vi "S2C_VLFT10_Proc_Read-WriteScales.vi"(8 "Error In":errorcluster, 10 "ScaleAction":u16(ring) items=["Read", "Write"], 11 "ScaleType":u16(ring) items=["Voltage", "Current"]) -> (0 "Error Out":errorcluster, 3 "Pass?":bool)   [LabVIEW 2015]
uses:
  Fornax/VIs/PolyDriver/S2C_FORNAX_Poly_ViperCmd.vi
panel:
  out "CurrSensScales":T1
  out "VoltSensScales":T2
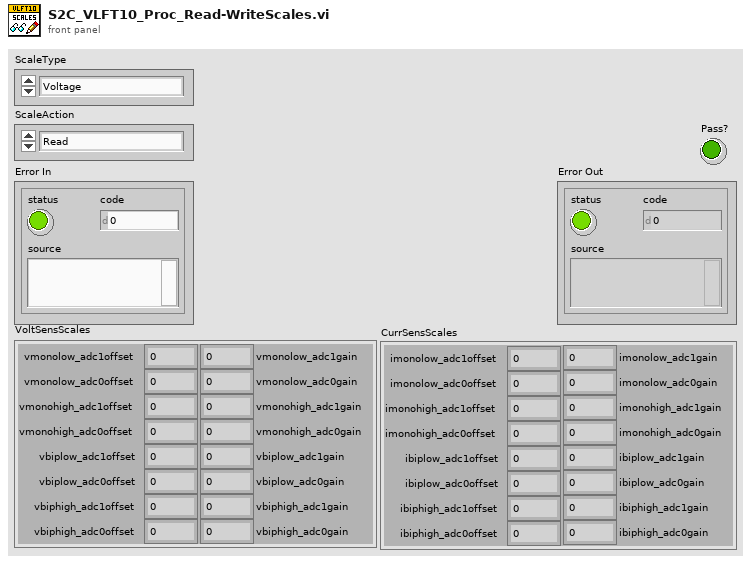
[diagram p1: front panel]
types:
  T1 = cluster{"imonolow_adc1offset":dbl, "imonolow_adc1gain":dbl, "imonolow_adc0offset":dbl, "imonolow_adc0gain":dbl, "imonohigh_adc1offset":dbl, "imonohigh_adc1gain":dbl, "imonohigh_adc0offset":dbl, "imonohigh_adc0gain":dbl, "ibiplow_adc1offset":dbl, "ibiplow_adc1gain":dbl, "ibiplow_adc0offset":dbl, "ibiplow_adc0gain":dbl, "ibiphigh_adc1offset":dbl, "ibiphigh_adc1gain":dbl, "ibiphigh_adc0offset":dbl, "ibiphigh_adc0gain":dbl}
  T2 = cluster{"vmonolow_adc1offset":dbl, "vmonolow_adc1gain":dbl, "vmonolow_adc0offset":dbl, "vmonolow_adc0gain":dbl, "vmonohigh_adc1offset":dbl, "vmonohigh_adc1gain":dbl, "vmonohigh_adc0offset":dbl, "vmonohigh_adc0gain":dbl, "vbiplow_adc1offset":dbl, "vbiplow_adc1gain":dbl, "vbiplow_adc0offset":dbl, "vbiplow_adc0gain":dbl, "vbiphigh_adc1offset":dbl, "vbiphigh_adc1gain":dbl, "vbiphigh_adc0offset":dbl, "vbiphigh_adc0gain":dbl}
  T3 = cluster{"Partition":string, "Message":string, "M_ViperMessage":string, "M_SrcId":i32}
  T4 = cluster{"vmonolow_adc0gain":dbl, "vmonolow_adc0offset":dbl, "vmonolow_adc1gain":dbl, "vmonolow_adc1offset":dbl, "vmonohigh_adc0gain":dbl, "vmonohigh_adc0offset":dbl, "vmonohigh_adc1gain":dbl, "vmonohigh_adc1offset":dbl, "vbiplow_adc0gain":dbl, "vbiplow_adc0offset":dbl, "vbiplow_adc1gain":dbl, "vbiplow_adc1offset":dbl, "vbiphigh_adc0gain":dbl, "vbiphigh_adc0offset":dbl, "vbiphigh_adc1gain":dbl, "vbiphigh_adc1offset":dbl}
  T5 = cluster{"Partition":string, "Message":string, "M_destId":i32, "M_message":string, "M_Crc32":i32}
  T6 = cluster{"imonolow_adc0gain":dbl, "imonolow_adc0offset":dbl, "imonolow_adc1gain":dbl, "imonolow_adc1offset":dbl, "imonohigh_adc0gain":dbl, "imonohigh_adc0offset":dbl, "imonohigh_adc1gain":dbl, "imonohigh_adc1offset":dbl, "ibiplow_adc0gain":dbl, "ibiplow_adc0offset":dbl, "ibiplow_adc1gain":dbl, "ibiplow_adc1offset":dbl, "ibiphigh_adc0gain":dbl, "ibiphigh_adc0offset":dbl, "ibiphigh_adc1gain":dbl, "ibiphigh_adc1offset":dbl}
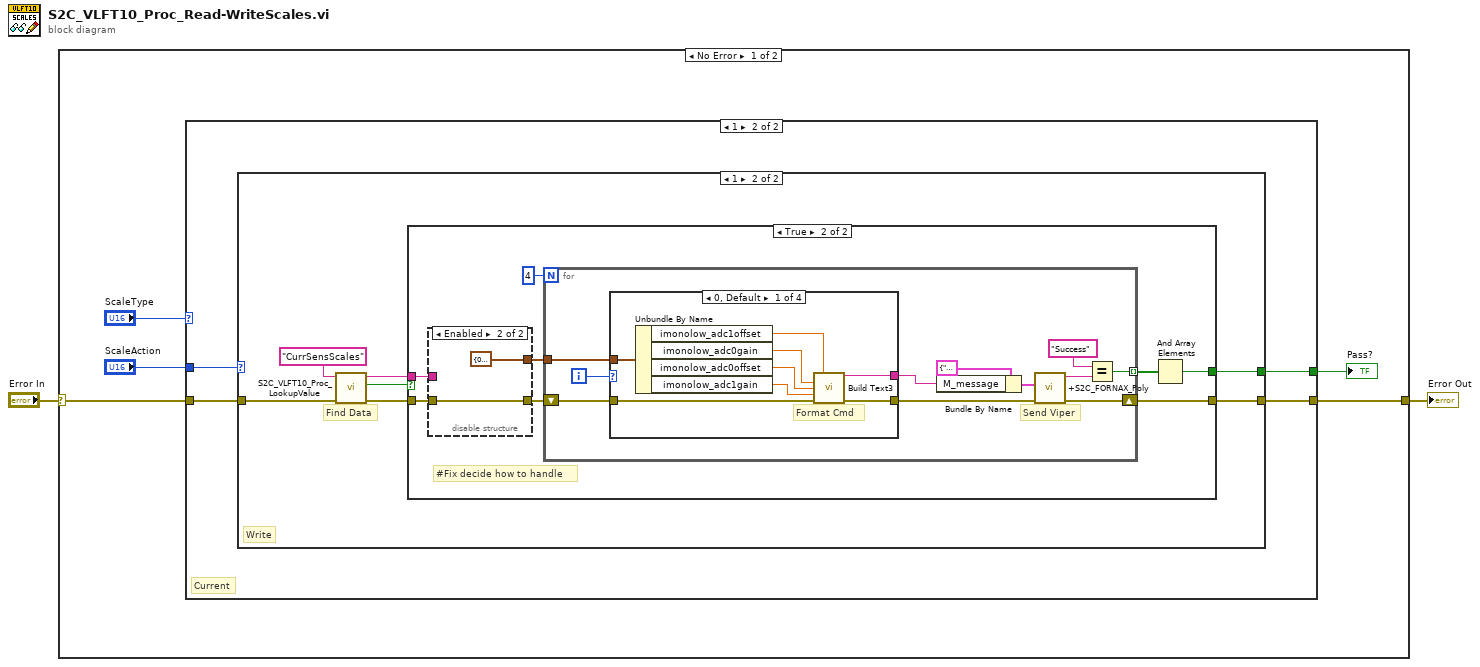
[diagram p0: block diagram]
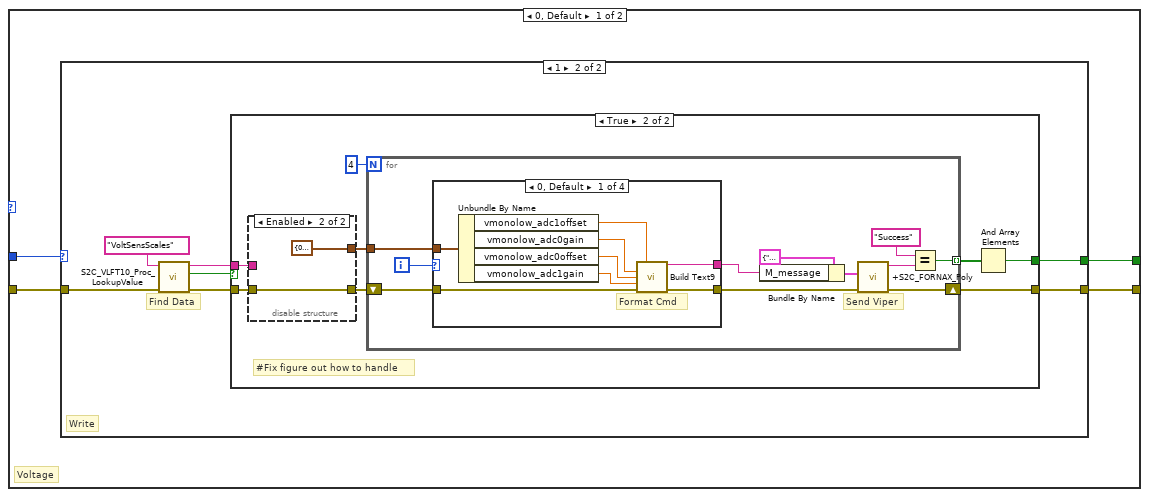
[diagram p2: hidden frame]
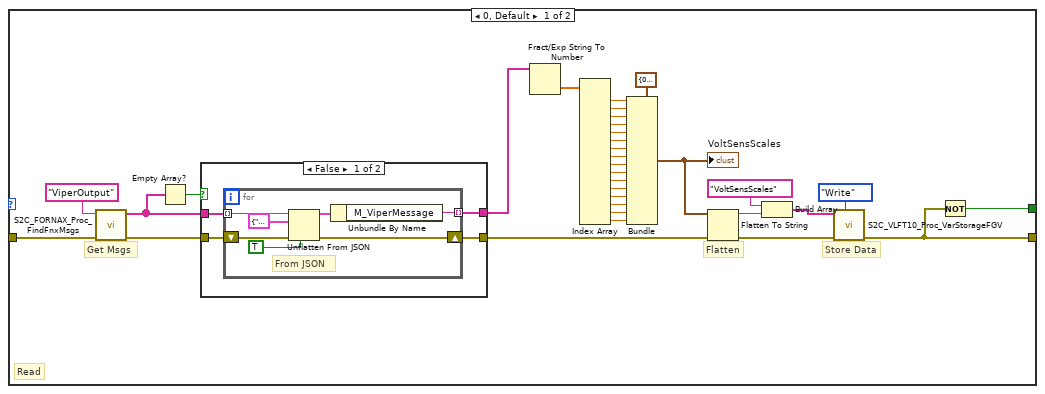
[diagram p3: hidden frame]
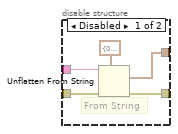
[diagram p6: hidden frame]
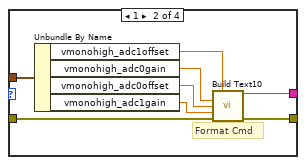
[diagram p7: hidden frame]
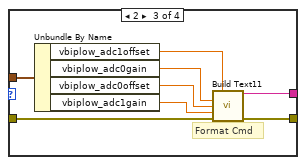
[diagram p8: hidden frame]
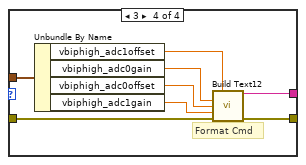
[diagram p9: hidden frame]
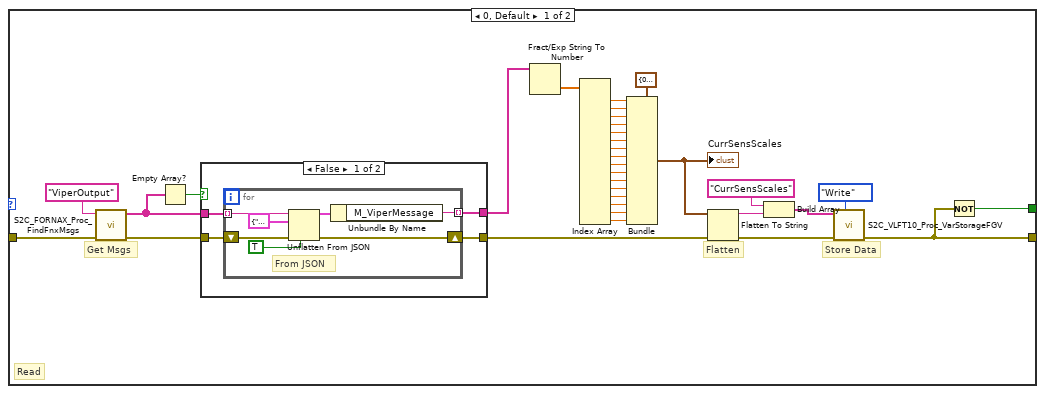
[diagram p10: hidden frame]
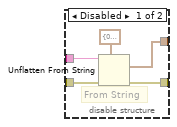
[diagram p13: hidden frame]
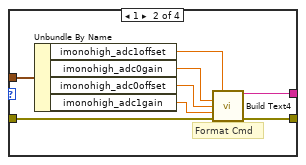
[diagram p14: hidden frame]
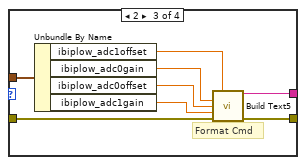
[diagram p15: hidden frame]
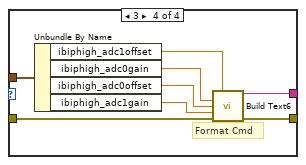
[diagram p16: hidden frame]
diagram:
  n1 = case shown="No Error" "Error In" {
    selector: "Error In" -> [w4 w238]
    tunnel: [w7 w238] -> w1
    frame No Error {
      n2 = case shown="1" "ScaleType" {
        tunnel: w4 -> [w11 w126]
        tunnel: [w10 w125] -> w7
        tunnel: "ScaleAction" -> [w9 w124]
        tunnel: [w8 w123] -> w3
        frame 0, Default {
          # "Voltage"
          n3 = case shown="1" w9 {
            tunnel: w11 -> [w14 w60]
            tunnel: [w13 w63] -> w10
            tunnel: [w12 w62] -> w8
            frame 0, Default {
              # "Flatten"
              # "Store Data"
              # "Read"
              # "Get Msgs"
              n4 = call "S2C_FORNAX_Proc_FindFnxMsgs.vi"("Error In"=w14, "MsgName"="ViperOutput") -> ("Error Out"=w43:errorcluster, "Messages"=w42:string[])  [unwired: 8 in]
              n5 = Empty Array?(array=w42) -> (empty?=w41:bool)
              n6 = case shown="False" w41 {
                tunnel: w43 -> [w48 w56]
                tunnel: w42 -> [w47 _]
                tunnel: [w45 w56] -> w15
                tunnel: [w46 _] -> w31
                frame False {
                  n7 = for {
                    tunnel: w47 -> [w52] mode=indexing
                    tunnel: [w50] -> w46 mode=indexing
                    shift-right: [w49] -> w45
                    shift-left: w48 -> [w54]
                    # "From JSON"
                    n8 = Unflatten From JSON(JSON string=w52, type and defaults=T3 {"Partition"="", "Message"="", "M_ViperMessage"="", "M_SrcId"=0}, default null elements? (F)=TRUE, error in (no error)=w54) -> (value=w51:T3, error out=w49:errorcluster)  [unwired: 3 in]
                    n9 = Unbundle By Name(w51) -> ("M_ViperMessage"=w50:string)
                  }
                }
                frame True {
                }
              }
              n10 = Fract/Exp String To Number(string=w31) -> (number=w40:dbl[])  [unwired: 3 in, 1 out]
              n11 = Index Array(array=w40) -> (element #1=w39:dbl, element #2=w38:dbl, element #3=w37:dbl, element #4=w36:dbl, element #5=w35:dbl, element #6=w34:dbl, element #7=w33:dbl, element #8=w32:dbl, element #9=w29:dbl, element #10=w28:dbl, element #11=w27:dbl, element #12=w26:dbl, element #13=w25:dbl, element #14=w24:dbl, element #15=w23:dbl, element #16=w22:dbl)  [unwired: 16 in]
              n12 = Bundle(cluster=T2 {"vmonolow_adc1offset"=0.0, "vmonolow_adc1gain"=0.0, "vmonolow_adc0offset"=0.0, "vmonolow_adc0gain"=0.0, "vmonohigh_adc1offset"=0.0, "vmonohigh_adc1gain"=0.0, "vmonohigh_adc0offset"=0.0, "vmonohigh_adc0gain"=0.0, "vbiplow_adc1offset"=0.0, "vbiplow_adc1gain"=0.0, "vbiplow_adc0offset"=0.0, "vbiplow_adc0gain"=0.0, "vbiphigh_adc1offset"=0.0, "vbiphigh_adc1gain"=0.0, "vbiphigh_adc0offset"=0.0, "vbiphigh_adc0gain"=0.0} ("VoltSensScales"), "vmonolow_adc1offset"=w39, "vmonolow_adc1gain"=w38, "vmonolow_adc0offset"=w37, "vmonolow_adc0gain"=w36, "vmonohigh_adc1offset"=w35, "vmonohigh_adc1gain"=w34, "vmonohigh_adc0offset"=w33, "vmonohigh_adc0gain"=w32, "vbiplow_adc1offset"=w29, "vbiplow_adc1gain"=w28, "vbiplow_adc0offset"=w27, "vbiplow_adc0gain"=w26, "vbiphigh_adc1offset"=w25, "vbiphigh_adc1gain"=w24, "vbiphigh_adc0offset"=w23, "vbiphigh_adc0gain"=w22) -> (w20:T2)
              "VoltSensScales" <- w20
              n13 = Flatten To String(anything=w20, error in (no error)=w15) -> (data string=w19:string, error out=w16:errorcluster)  [unwired: 2 in, 1 out]
              n14 = Build Array("VoltSensScales", w19) -> (w17:string[])
              n15 = call "S2C_VLFT10_Proc_VarStorageFGV.vi"("Action"=enum16{"Read", "Write", "Clear"}."Write", "Error In"=w16, "Data In"=w17) -> ("Error Out"=w13:errorcluster)  [unwired: 7 in, 1 out]
              n16 = Not(x=w13) -> (.not. x?=w12:bool)
            }
            frame 1 {
              # "Write"
              # "Find Data"
              n17 = call "S2C_VLFT10_Proc_LookupValue.vi"("Error In"=w60, "VarName"="VoltSensScales") -> ("Error Out"=w59:errorcluster, "Found?"=w57:bool, "VarValue"=w58:string)  [unwired: 7 in]
              n18 = case shown="True" w57 {
                tunnel: w58 -> [_ w67]
                tunnel: w59 -> [w64 w68]
                tunnel: [w64 w65] -> w63
                tunnel: [_ w72] -> w62
                frame False {
                }
                frame True {
                  # "#Fix figure out how to handle"
                  n19 = disable-structure shown="Enabled" {
                    disable-tunnel: [w77 w79] -> w70
                    disable-tunnel: [w76 T2 {"vmonolow_adc1offset"=0.0, "vmonolow_adc1gain"=1.0, "vmonolow_adc0offset"=0.0, "vmonolow_adc0gain"=1.0, "vmonohigh_adc1offset"=0.0, "vmonohigh_adc1gain"=1.0, "vmonohigh_adc0offset"=0.0, "vmonohigh_adc0gain"=1.0, "vbiplow_adc1offset"=0.0, "vbiplow_adc1gain"=1.0, "vbiplow_adc0offset"=0.0, "vbiplow_adc0gain"=1.0, "vbiphigh_adc1offset"=0.0, "vbiphigh_adc1gain"=1.0, "vbiphigh_adc0offset"=0.0, "vbiphigh_adc0gain"=1.0} ("VoltSensScales 2")] -> w69
                    disable-tunnel: w68 -> [w75 w79]
                    disable-tunnel: w67 -> [w74 _]
                    frame Disabled {
                      # "From String"
                      n20 = Unflatten From String(type=T4 {"vmonolow_adc0gain"=0.0, "vmonolow_adc0offset"=0.0, "vmonolow_adc1gain"=0.0, "vmonolow_adc1offset"=0.0, "vmonohigh_adc0gain"=0.0, "vmonohigh_adc0offset"=0.0, "vmonohigh_adc1gain"=0.0, "vmonohigh_adc1offset"=0.0, "vbiplow_adc0gain"=0.0, "vbiplow_adc0offset"=0.0, "vbiplow_adc1gain"=0.0, "vbiplow_adc1offset"=0.0, "vbiphigh_adc0gain"=0.0, "vbiphigh_adc0offset"=0.0, "vbiphigh_adc1gain"=0.0, "vbiphigh_adc1offset"=0.0} ("Sensor Global Scales"), binary string=w74, error in (no error)=w75) -> (value=w76:T4, error out=w77:errorcluster)  [unwired: 2 in, 1 out]
                    }
                    frame Enabled {
                    }
                  }
                  n21 = for {
                    N: 4 -> [_]
                    tunnel: w69 -> [w85]
                    shift-right: [w90] -> w65
                    shift-left: w70 -> [w88]
                    tunnel: [w89] -> w66 mode=indexing
                    i -> [w84]
                    # "Send Viper"
                    n22 = case shown="0, Default" w84 {
                      tunnel: w85 -> [w98 w106 w114 w122]
                      tunnel: w88 -> [w93 w101 w109 w117]
                      tunnel: [w92 w100 w108 w116] -> w87
                      tunnel: [w91 w99 w107 w115] -> w86
                      frame 0, Default {
                        # "Format Cmd"
                        n23 = Unbundle By Name(w98) -> ("vmonolow_adc1offset"=w94:dbl, "vmonolow_adc0gain"=w95:dbl, "vmonolow_adc0offset"=w96:dbl, "vmonolow_adc1gain"=w97:dbl)
                        n24 = call "Build Text9"("vMonoLow1Offset"=w94, "vMonoLow0Gain"=w95, "vMonoLow0Offset"=w96, "vMonoLow1Gain"=w97, "error in (no error)"=w93) -> ("Result"=w91:string, "error out"=w92:errorcluster)  [unwired: 9 in]
                      }
                      frame 1 {
                        # "Format Cmd"
                        n25 = Unbundle By Name(w106) -> ("vmonohigh_adc1offset"=w102:dbl, "vmonohigh_adc0gain"=w103:dbl, "vmonohigh_adc0offset"=w104:dbl, "vmonohigh_adc1gain"=w105:dbl)
                        n26 = call "Build Text10"("vMonoHigh1Offset"=w102, "vMonoHigh0Gain"=w103, "vMonoHigh0Offset"=w104, "vMonoHigh1Gain"=w105, "error in (no error)"=w101) -> ("Result"=w99:string, "error out"=w100:errorcluster)  [unwired: 9 in]
                      }
                      frame 2 {
                        # "Format Cmd"
                        n27 = Unbundle By Name(w114) -> ("vbiplow_adc1offset"=w110:dbl, "vbiplow_adc0gain"=w111:dbl, "vbiplow_adc0offset"=w112:dbl, "vbiplow_adc1gain"=w113:dbl)
                        n28 = call "Build Text11"("vBipLow1Offset"=w110, "vBipLow0Gain"=w111, "BipLow0Offset"=w112, "vBipLow1Gain"=w113, "error in (no error)"=w109) -> ("Result"=w107:string, "error out"=w108:errorcluster)  [unwired: 9 in]
                      }
                      frame 3 {
                        # "Format Cmd"
                        n29 = Unbundle By Name(w122) -> ("vbiphigh_adc1offset"=w118:dbl, "vbiphigh_adc0gain"=w119:dbl, "vbiphigh_adc0offset"=w120:dbl, "vbiphigh_adc1gain"=w121:dbl)
                        n30 = call "Build Text12"("vBipHigh1Offset"=w118, "vBipHigh0Gain"=w119, "vBipHigh0Offset"=w120, "vBipHigh1Gain"=w121, "error in (no error)"=w117) -> ("Result"=w115:string, "error out"=w116:errorcluster)  [unwired: 9 in]
                      }
                    }
                    n31 = Bundle By Name(cluster=T5 {"Partition"="Default", "Message"="ViperInput", "M_destId"=1, "M_message"="", "M_Crc32"=0} ("ViperCmd"), "M_message"=w86) -> (w82:T5)
                    n32 = call-poly "+S2C_FORNAX_Poly.vi"("Error In"=w87, "ViperCmd"=w82) -> ("Error Out"=w90:errorcluster, "Response"=w81:string)  [unwired: 8 in]
                    n33 = Equal?(x="Success", y=w81) -> (x = y?=w89:bool)
                  }
                  n34 = And Array Elements(Boolean array=w66) -> (logical AND=w72:bool)
                }
              }
            }
          }
        }
        frame 1 {
          # "Current"
          n35 = case shown="1" w124 {
            tunnel: w126 -> [w139 w175]
            tunnel: [w138 w174] -> w125
            tunnel: [w137 w173] -> w123
            frame 0, Default {
              # "Flatten"
              # "Store Data"
              # "Get Msgs"
              # "Read"
              n36 = call "S2C_FORNAX_Proc_FindFnxMsgs.vi"("Error In"=w139, "MsgName"="ViperOutput") -> ("Error Out"=w158:errorcluster, "Messages"=w157:string[])  [unwired: 8 in]
              n37 = Empty Array?(array=w157) -> (empty?=w156:bool)
              n38 = case shown="False" w156 {
                tunnel: w158 -> [w163 w171]
                tunnel: w157 -> [w162 _]
                tunnel: [w160 w171] -> w140
                tunnel: [w161 _] -> w146
                frame False {
                  n39 = for {
                    tunnel: w162 -> [w167] mode=indexing
                    tunnel: [w165] -> w161 mode=indexing
                    shift-right: [w164] -> w160
                    shift-left: w163 -> [w169]
                    # "From JSON"
                    n40 = Unflatten From JSON(JSON string=w167, type and defaults=T3 {"Partition"="", "Message"="", "M_ViperMessage"="", "M_SrcId"=0}, default null elements? (F)=TRUE, error in (no error)=w169) -> (value=w166:T3, error out=w164:errorcluster)  [unwired: 3 in]
                    n41 = Unbundle By Name(w166) -> ("M_ViperMessage"=w165:string)
                  }
                }
                frame True {
                }
              }
              n42 = Fract/Exp String To Number(string=w146) -> (number=w155:dbl[])  [unwired: 3 in, 1 out]
              n43 = Index Array(array=w155) -> (element #1=w154:dbl, element #2=w153:dbl, element #3=w152:dbl, element #4=w151:dbl, element #5=w150:dbl, element #6=w149:dbl, element #7=w148:dbl, element #8=w147:dbl, element #9=w128:dbl, element #10=w129:dbl, element #11=w130:dbl, element #12=w131:dbl, element #13=w132:dbl, element #14=w133:dbl, element #15=w134:dbl, element #16=w135:dbl)  [unwired: 16 in]
              n44 = Bundle(cluster=T1 {"imonolow_adc1offset"=0.0, "imonolow_adc1gain"=0.0, "imonolow_adc0offset"=0.0, "imonolow_adc0gain"=0.0, "imonohigh_adc1offset"=0.0, "imonohigh_adc1gain"=0.0, "imonohigh_adc0offset"=0.0, "imonohigh_adc0gain"=0.0, "ibiplow_adc1offset"=0.0, "ibiplow_adc1gain"=0.0, "ibiplow_adc0offset"=0.0, "ibiplow_adc0gain"=0.0, "ibiphigh_adc1offset"=0.0, "ibiphigh_adc1gain"=0.0, "ibiphigh_adc0offset"=0.0, "ibiphigh_adc0gain"=0.0} ("Sensor Global Scales"), "imonolow_adc1offset"=w154, "imonolow_adc1gain"=w153, "imonolow_adc0offset"=w152, "imonolow_adc0gain"=w151, "imonohigh_adc1offset"=w150, "imonohigh_adc1gain"=w149, "imonohigh_adc0offset"=w148, "imonohigh_adc0gain"=w147, "ibiplow_adc1offset"=w128, "ibiplow_adc1gain"=w129, "ibiplow_adc0offset"=w130, "ibiplow_adc0gain"=w131, "ibiphigh_adc1offset"=w132, "ibiphigh_adc1gain"=w133, "ibiphigh_adc0offset"=w134, "ibiphigh_adc0gain"=w135) -> (w127:T1)
              "CurrSensScales" <- w127
              n45 = Flatten To String(anything=w127, error in (no error)=w140) -> (data string=w144:string, error out=w141:errorcluster)  [unwired: 2 in, 1 out]
              n46 = Build Array("CurrSensScales", w144) -> (w142:string[])
              n47 = call "S2C_VLFT10_Proc_VarStorageFGV.vi"("Action"=enum16{"Read", "Write", "Clear"}."Write", "Error In"=w141, "Data In"=w142) -> ("Error Out"=w138:errorcluster)  [unwired: 7 in, 1 out]
              n48 = Not(x=w138) -> (.not. x?=w137:bool)
            }
            frame 1 {
              # "Find Data"
              # "Write"
              n49 = call "S2C_VLFT10_Proc_LookupValue.vi"("Error In"=w175, "VarName"="CurrSensScales") -> ("Error Out"=w177:errorcluster, "Found?"=w172:bool, "VarValue"=w178:string)  [unwired: 7 in]
              n50 = case shown="True" w172 {
                tunnel: w178 -> [_ w182]
                tunnel: w177 -> [w179 w183]
                tunnel: [w179 w180] -> w174
                tunnel: [_ w187] -> w173
                frame False {
                }
                frame True {
                  # "#Fix decide how to handle"
                  n51 = disable-structure shown="Enabled" {
                    disable-tunnel: [w191 w193] -> w185
                    disable-tunnel: [w190 T1 {"imonolow_adc1offset"=0.0, "imonolow_adc1gain"=1.0, "imonolow_adc0offset"=0.0, "imonolow_adc0gain"=1.0, "imonohigh_adc1offset"=0.0, "imonohigh_adc1gain"=1.0, "imonohigh_adc0offset"=0.0, "imonohigh_adc0gain"=1.0, "ibiplow_adc1offset"=0.0, "ibiplow_adc1gain"=1.0, "ibiplow_adc0offset"=0.0, "ibiplow_adc0gain"=1.0, "ibiphigh_adc1offset"=0.0, "ibiphigh_adc1gain"=1.0, "ibiphigh_adc0offset"=0.0, "ibiphigh_adc0gain"=1.0} ("CurrSensScales 2")] -> w184
                    disable-tunnel: w183 -> [w189 w193]
                    disable-tunnel: w182 -> [w188 _]
                    frame Disabled {
                      # "From String"
                      n52 = Unflatten From String(type=T6 {"imonolow_adc0gain"=0.0, "imonolow_adc0offset"=0.0, "imonolow_adc1gain"=0.0, "imonolow_adc1offset"=0.0, "imonohigh_adc0gain"=0.0, "imonohigh_adc0offset"=0.0, "imonohigh_adc1gain"=0.0, "imonohigh_adc1offset"=0.0, "ibiplow_adc0gain"=0.0, "ibiplow_adc0offset"=0.0, "ibiplow_adc1gain"=0.0, "ibiplow_adc1offset"=0.0, "ibiphigh_adc0gain"=0.0, "ibiphigh_adc0offset"=0.0, "ibiphigh_adc1gain"=0.0, "ibiphigh_adc1offset"=0.0} ("Sensor Global Scales"), binary string=w188, error in (no error)=w189) -> (value=w190:T6, error out=w191:errorcluster)  [unwired: 2 in, 1 out]
                    }
                    frame Enabled {
                    }
                  }
                  n53 = for {
                    N: 4 -> [_]
                    tunnel: w184 -> [w205]
                    shift-right: [w200] -> w180
                    shift-left: w185 -> [w204]
                    tunnel: [w199] -> w181 mode=indexing
                    i -> [w203]
                    # "Send Viper"
                    n54 = case shown="0, Default" w203 {
                      tunnel: w205 -> [w213 w221 w229 w237]
                      tunnel: w204 -> [w208 w216 w224 w232]
                      tunnel: [w207 w215 w223 w231] -> w202
                      tunnel: [w206 w214 w222 w230] -> w201
                      frame 0, Default {
                        # "Format Cmd"
                        n55 = Unbundle By Name(w213) -> ("imonolow_adc1offset"=w209:dbl, "imonolow_adc0gain"=w210:dbl, "imonolow_adc0offset"=w211:dbl, "imonolow_adc1gain"=w212:dbl)
                        n56 = call "Build Text3"("iMonoLow1Offset"=w209, "iMonoLow0Gain"=w210, "iMonoLow0Offset"=w211, "iMonoLow1Gain"=w212, "error in (no error)"=w208) -> ("Result"=w206:string, "error out"=w207:errorcluster)  [unwired: 9 in]
                      }
                      frame 1 {
                        # "Format Cmd"
                        n57 = Unbundle By Name(w221) -> ("imonohigh_adc1offset"=w217:dbl, "imonohigh_adc0gain"=w218:dbl, "imonohigh_adc0offset"=w219:dbl, "imonohigh_adc1gain"=w220:dbl)
                        n58 = call "Build Text4"("iMonoHigh1Offset"=w217, "iMonoHigh0Gain"=w218, "iMonoHigh0Offset"=w219, "iMonoHigh1Gain"=w220, "error in (no error)"=w216) -> ("Result"=w214:string, "error out"=w215:errorcluster)  [unwired: 9 in]
                      }
                      frame 2 {
                        # "Format Cmd"
                        n59 = Unbundle By Name(w229) -> ("ibiplow_adc1offset"=w225:dbl, "ibiplow_adc0gain"=w226:dbl, "ibiplow_adc0offset"=w227:dbl, "ibiplow_adc1gain"=w228:dbl)
                        n60 = call "Build Text5"("iBipLow1Offset"=w225, "iBipLow0Gain"=w226, "iBipLow0Offset"=w227, "iBipLow1Gain"=w228, "error in (no error)"=w224) -> ("Result"=w222:string, "error out"=w223:errorcluster)  [unwired: 9 in]
                      }
                      frame 3 {
                        # "Format Cmd"
                        n61 = Unbundle By Name(w237) -> ("ibiphigh_adc1offset"=w233:dbl, "ibiphigh_adc0gain"=w234:dbl, "ibiphigh_adc0offset"=w235:dbl, "ibiphigh_adc1gain"=w236:dbl)
                        n62 = call "Build Text6"("iBipHigh1Offset"=w233, "iBipHigh0Gain"=w234, "iBipHigh0Offset"=w235, "iBipHigh1Gain"=w236, "error in (no error)"=w232) -> ("Result"=w230:string, "error out"=w231:errorcluster)  [unwired: 9 in]
                      }
                    }
                    n63 = Bundle By Name(cluster=T5 {"Partition"="Default", "Message"="ViperInput", "M_destId"=1, "M_message"="", "M_Crc32"=0} ("ViperCmd"), "M_message"=w201) -> (w197:T5)
                    n64 = call-poly "+S2C_FORNAX_Poly.vi"("Error In"=w202, "ViperCmd"=w197) -> ("Error Out"=w200:errorcluster, "Response"=w196:string)  [unwired: 8 in]
                    n65 = Equal?(x="Success", y=w196) -> (x = y?=w199:bool)
                  }
                  n66 = And Array Elements(Boolean array=w181) -> (logical AND=w187:bool)
                }
              }
            }
          }
        }
      }
      "Pass?" <- w3
    }
    frame Error {
    }
  }
  "Error Out" <- w1
